vi "GetClassName.vi"(8 "error in (no error)":errorcluster, 11 "object":refnum<class>) -> (0 "error out":errorcluster, 3 "Class Name":string)   [LabVIEW 2020]
uses:
  <vilib>/regexp/Match Regular Expression.xnode
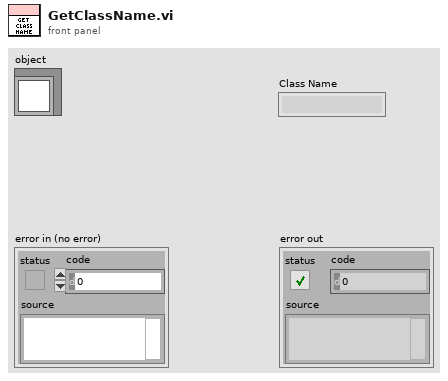
[diagram p1: front panel]
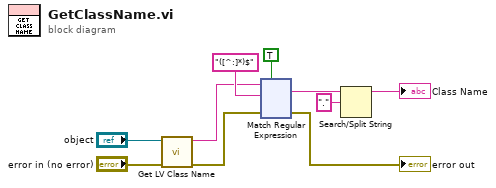
[diagram p0: block diagram]
diagram:
  n1 = call <vilib>:"Get LV Class Name.vi"("error in (no error)"="error in (no error)", "object"="object") -> ("error out"=w9:errorcluster, "class name"=w6:string)  [unwired: 8 in]
  n2 = xnode "Match Regular Expression"("input string"=w6, "regular expression"="([^:]*)$", "error in"=w9, "ignore case? (F)"=TRUE) -> ("whole match"=w5:string, "error out"=→"error out":errorcluster)  [unwired: 2 in, 3 out]
  n3 = Search/Split String(string=w5, search string/char (-)=".") -> (substring before match=→"Class Name":string)  [unwired: 1 in, 2 out]
